vi "XSP3_Get_Data_v2.vi"(3 "offset_roi":i32[][](array[numeric]), 5 "offset_icr":i32[](array[numeric]), 7 "1st ch":i32=1, 8 "ErrorIn":errorcluster, 9 "num point":i32=1, 10 "num roi":i32=1, 11 "num ch":i32=8) -> (0 "ErrorOut":errorcluster, 1 "save data":dbl[][](array[numeric]), 2 "roi sum":dbl[][](array[numeric]), 4 "RoiData":dbl[][][](array[numeric]) format="%.2f", 6 "IcrData":dbl[][](array[numeric]) format="%.2f")   [LabVIEW 2010]
panel:
  in  "ミリ秒倍数":u32
  # "ch"
  # "point"
  # "roi"
  # "ch"
  # "point"
  # "roi"
  # "ch"
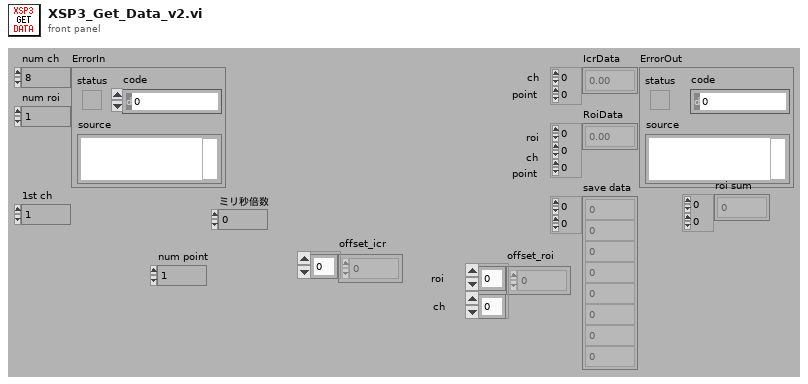
[diagram p1: front panel]
types:
  T1 = cluster{"MCA":dbl[][], "MCAsum":dbl[][], "ROI/ICRlast":dbl[], "ROI/ICRarray":dbl[][], "DeadTime":dbl[]}
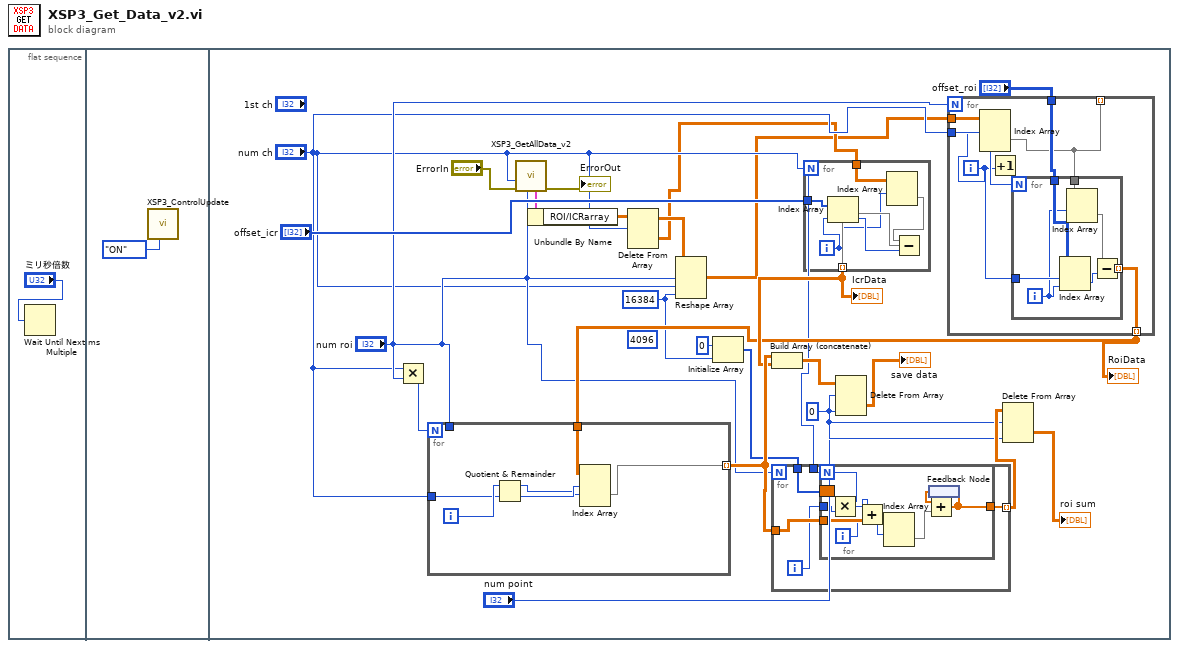
[diagram p0: block diagram]
diagram:
  n1 = flat-sequence {
    frame #0 {
      n2 = Wait Until Next ms Multiple(millisecond multiple="ミリ秒倍数") -> ()  [unwired: 1 out]
    }
    frame #1 {
      n3 = call "XSP3_ControlUpdate.vi"("Erase"=enum16{"OFF", "ON"}."ON") -> ()  [unwired: 8 in, 3 out]
    }
    frame #2 {
      (unwired) 4096 ("dimension size")
      w3 = 16384 ("dimension size")
      w19 = 0 ("無効な指標 （列）")
      n4 = Multiply(x="num ch", y="num roi") -> (x*y=w26:i32)
      n5 = call "XSP3_GetAllData_v2.vi"("NumRoi"="num roi", "ErrorIn"="ErrorIn", "NumCh"="num ch") -> ("ErrorOut"=→"ErrorOut":errorcluster, "Data"=w12:T1)  [unwired: 5 in, 2 out]
      n6 = Unbundle By Name(w12) -> ("ROI/ICRarray"=w11:dbl[][])
      n7 = Delete From Array(array=w11, length="num ch") -> (deleted portion=w7:dbl[][], array with subset deleted=w10:dbl[][])  [unwired: 2 in]
      n8 = Reshape Array(w10, "num roi", "num ch", w3) -> (w5:dbl[][][])
      n9 = Initialize Array(0 ("要素"), w3) -> (w21:i32[])
      n10 = for {
        N: "num ch" -> [_]
        tunnel: "offset_icr" -> [w42]
        tunnel: w7 -> [w44]
        tunnel: [w45] -> w15 mode=indexing
        i -> [w40]
        n11 = Index Array(array=w42, index=w40) -> (element=w43:i32)
        n12 = Index Array(array=w44, index (row)=w40) -> (element=w41:dbl[])  [unwired: 1 in]
        n13 = Subtract(x=w41, y=w43) -> (x-y=w45:dbl[])
      }
      "IcrData" <- w15
      n14 = for {
        N: "num roi" -> [_]
        tunnel: "num ch" -> [w30]
        tunnel: "offset_roi" -> [w32]
        tunnel: [w31] -> w13 mode=indexing
        tunnel: [w27] -> _ mode=indexing
        tunnel: w5 -> [w29]
        i -> [w28]
        n15 = Index Array(array=w29, index (dim 0)=w28) -> (element=w27:dbl[][])  [unwired: 2 in]
        n16 = Increment(x=w28) -> ()  [unwired: 1 out]
        n17 = for {
          N: w30 -> [_]
          tunnel: w32 -> [w39]
          tunnel: w28 -> [w36]
          tunnel: [w37] -> w31 mode=indexing
          tunnel: w27 -> [w35]
          i -> [w33]
          n18 = Index Array(array=w39, index (row)=w36, index (col)=w33) -> (element=w38:i32)
          n19 = Index Array(array=w35, index (row)=w33) -> (element=w34:dbl[])  [unwired: 1 in]
          n20 = Subtract(x=w34, y=w38) -> (x-y=w37:dbl[])
        }
      }
      "RoiData" <- w13
      n21 = for {
        N: w26 -> [_]
        tunnel: w13 -> [w65]
        tunnel: [w64] -> w23 mode=indexing
        tunnel: "num roi" -> [_]
        tunnel: "num ch" -> [w62]
        i -> [w63]
        n22 = Quotient & Remainder(x=w63, y=w62) -> (x-y*floor(x/y)=w60:i32, floor(x/y)=w61:i32)
        n23 = Index Array(array=w65, index (dim 0)=w61, index (dim 1)=w60) -> (element=w64:dbl[])  [unwired: 1 in]
      }
      n24 = Build Array (concatenate)(w23, w15) -> (w25:dbl[][])
      n25 = for {
        N: "num roi" -> [_]
        tunnel: w23 -> [w49]
        tunnel: "num ch" -> [w50]
        tunnel: [w47] -> w20 mode=indexing
        tunnel: w21 -> [w46]
        i -> [w48]
        n26 = for {
          N: w50 -> [w58]
          tunnel: w49 -> [w59]
          tunnel: w48 -> [w57]
          border: w46 -> [_]
          tunnel: [w52] -> w47
          i -> [w55]
          n27 = Multiply(x=w58, y=w57) -> (x*y=w56:i32)
          n28 = Add(x=w56, y=w55) -> (x+y=w51:i32)
          n29 = Index Array(array=w59, index (row)=w51) -> (element=w54:dbl[])  [unwired: 1 in]
          n30 = feedback #1() -> (w53:dbl[])
          n31 = Add(x=w53, y=w54) -> (x+y=w52:dbl[])
          n32 = feedback-in #1(w52) -> ()
        }
      }
      n33 = Delete From Array(array=w25, length="num point", index (col)=w19) -> (deleted portion=→"save data":dbl[][])  [unwired: 1 in, 1 out]
      n34 = Delete From Array(array=w20, length="num point", index (col)=w19) -> (deleted portion=→"roi sum":dbl[][])  [unwired: 1 in, 1 out]
    }
  }
